vi "LV to ITX 2D AutoPlot.vi"(0 "filename":string, 1 "path":path, 5 "Notes":string, 7 "2D Array":dbl[][](array[numeric]), 9 "X, Y Arrays":cluster{"X 1D Array":dbl[], "Y 1D Array":dbl[]}={"X 1D Array"=[0.0, 1.0], "Y 1D Array"=[0.0, 1.0]}, 11 "X, Y wavenames":string[](array[string])=["x_", "y_"], 12 "X,Y,Z Labels":string[](array[string])=["x", "y"], 14 "input command string":string="Display;AppendImage '#wave2D#'\nModifyGraph width=216,height={Aspect,1}\nLabel bottom \"#labelX#\"\nLabel left \"#labelY#\"\nModifyImage '#wave2D#' ctab= {*,*,Rainbow,1}\nModifyGraph mirror=1") -> (4 "file":path)   [LabVIEW 2016, in "LVtoITX.lvclass"]
doc: "Write your 2D data to ITX file. This AutoPlot VI adds commands that will automatically create in Igor an intensity graph with X and Y axes scaled by the 1D arrays, allowing you to quickly view your data.\n\n-- path: base path to save data\n-- filename: base filename\n-- Notes: add any notes here to help you remember what experiment you did\n-- 2D Array: Intensity data\n-- X,Y Arrays: These are used to apply an appropriate scaling to the intensity graph\n-- X,Y wavenames: Default \"x_\" and \"y_\" are fine.\n-- X,Y,Z Labels: Labels for plotting in Igor."
uses:
  LVtoITX.lvclass
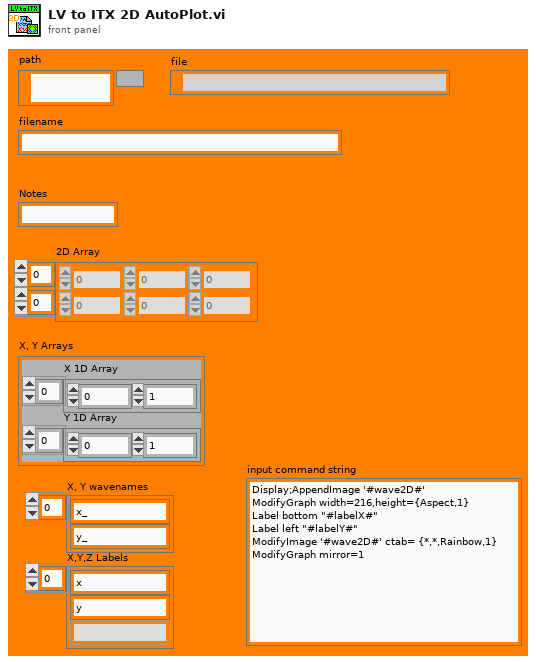
[diagram p1: front panel]
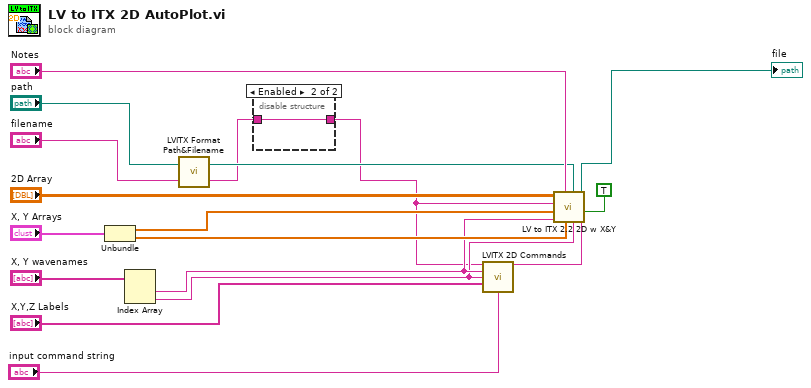
[diagram p0: block diagram]
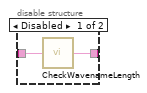
[diagram p2: hidden frame]
diagram:
  n1 = Unbundle("X, Y Arrays") -> ("X 1D Array"=w13:dbl[], "Y 1D Array"=w12:dbl[])
  n2 = Index Array(array="X, Y wavenames") -> (element #1=w9:string, element #2=w8:string)  [unwired: 2 in]
  n3 = call "LVITX Format Path&Filename.vi"("filename"="filename", "path"="path") -> ("file name without extension"=w3:string, "dup file"=w14:path)
  n4 = disable-structure shown="Enabled" {
    disable-tunnel: w3 -> [w20 w21]
    disable-tunnel: [w19 w21] -> w2
    frame Disabled {
      n5 = call "CheckWavenameLength.vi"("wavename"=w20) -> ("wavename"=w19:string)
    }
    frame Enabled {
    }
  }
  n6 = call "LVITX 2D Commands.vi"("2D wavename"=w2, "X wavename"=w9, "Y wavename"=w8, "X,Y,Z Labels"="X,Y,Z Labels", "input string"="input command string") -> ("result string"=w5:string)  [unwired: 1 in, 9 out]
  n7 = call "LV to ITX 2.2 2D w X&Y.vi"("Commands"=w5, "Kill X&Y waves?"=TRUE, "Y Array name"=w8, "filename"=w14, "Y 1D Array"=w12, "Notes"="Notes", "X  Array name"=w9, "X 1D Array"=w13, "2D Array name"=w2, "2D Array"="2D Array") -> ("file"=→"file":path)  [unwired: 1 out]
